vi "FinalizeListGeneration.vi"(8 "error in (no error)":errorcluster, 9 "Root path":path, 10 "CDependencyList in":refnum<class "CDependencyList.lvclass">, 11 "CReporter in":refnum<class "CReporter.lvclass">) -> (0 "error out":errorcluster, 3 "CReporter out":refnum<class "CReporter.lvclass">)   [LabVIEW 2020, in "DependencyInspection.lvlib" / "CReporter.lvclass"]
uses:
  CReporter.lvclass
  CDependencyList/CDependencyList.lvclass
  CReporter.lvclass/CReporter.ctl
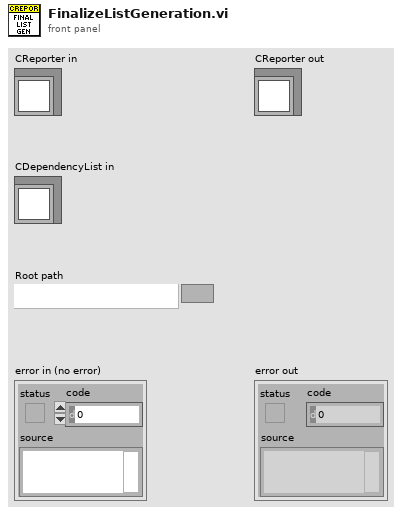
[diagram p1: front panel]
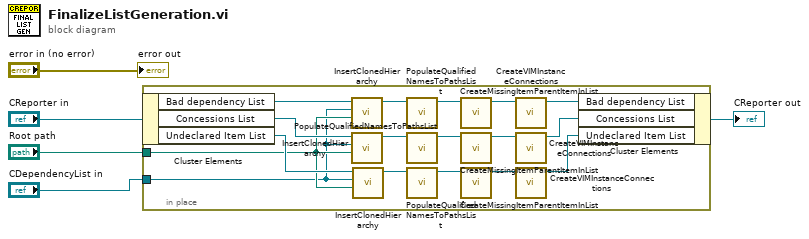
[diagram p0: block diagram]
diagram:
  n1 = in-place {
    in-place-border: "Root path" -> [w7]
    in-place-border: "CDependencyList in" -> [w6]
    n2 = in-place-cluster #1("CReporter in") -> ("Bad dependency List"=w13:refnum<class "CDependencyList.lvclass">, "Concessions List"=w11:refnum<class "CDependencyList.lvclass">, "Undeclared Item List"=w9:refnum<class "CDependencyList.lvclass">)
    n3 = call-dynamic "InsertClonedHierarchy.vi"("Root path"=w7, "Dependency List in"=w6, "CDependencyList in"=w13) -> ("CDependencyList out"=w12:refnum<class "CDependencyList.lvclass">)  [unwired: 7 in, 1 out]
    n4 = call-dynamic "InsertClonedHierarchy.vi"("Root path"=w7, "Dependency List in"=w6, "CDependencyList in"=w11) -> ("CDependencyList out"=w10:refnum<class "CDependencyList.lvclass">)  [unwired: 7 in, 1 out]
    n5 = call-dynamic "InsertClonedHierarchy.vi"("Root path"=w7, "Dependency List in"=w6, "CDependencyList in"=w9) -> ("CDependencyList out"=w8:refnum<class "CDependencyList.lvclass">)  [unwired: 7 in, 1 out]
    n6 = call-dynamic "PopulateQualifiedNamesToPathsList.vi"("CDependencyList in"=w12) -> ("CDependencyList out"=w21:refnum<class "CDependencyList.lvclass">)  [unwired: 9 in, 1 out]
    n7 = call-dynamic "PopulateQualifiedNamesToPathsList.vi"("CDependencyList in"=w10) -> ("CDependencyList out"=w19:refnum<class "CDependencyList.lvclass">)  [unwired: 9 in, 1 out]
    n8 = call-dynamic "PopulateQualifiedNamesToPathsList.vi"("CDependencyList in"=w8) -> ("CDependencyList out"=w17:refnum<class "CDependencyList.lvclass">)  [unwired: 9 in, 1 out]
    n9 = call-dynamic "CreateMissingItemParentItemInList.vi"("CDependencyList in"=w21) -> ("CDependencyList out"=w22:refnum<class "CDependencyList.lvclass">)  [unwired: 9 in, 1 out]
    n10 = call-dynamic "CreateMissingItemParentItemInList.vi"("CDependencyList in"=w19) -> ("CDependencyList out"=w20:refnum<class "CDependencyList.lvclass">)  [unwired: 9 in, 1 out]
    n11 = call-dynamic "CreateMissingItemParentItemInList.vi"("CDependencyList in"=w17) -> ("CDependencyList out"=w18:refnum<class "CDependencyList.lvclass">)  [unwired: 9 in, 1 out]
    n12 = call-dynamic "CreateVIMInstanceConnections.vi"("CDependencyList in"=w22) -> ("CDependencyList out"=w16:refnum<class "CDependencyList.lvclass">)  [unwired: 9 in, 1 out]
    n13 = call-dynamic "CreateVIMInstanceConnections.vi"("CDependencyList in"=w20) -> ("CDependencyList out"=w15:refnum<class "CDependencyList.lvclass">)  [unwired: 9 in, 1 out]
    n14 = call-dynamic "CreateVIMInstanceConnections.vi"("CDependencyList in"=w18) -> ("CDependencyList out"=w14:refnum<class "CDependencyList.lvclass">)  [unwired: 9 in, 1 out]
    n15 = in-place-cluster #1("Bad dependency List"=w16, "Concessions List"=w15, "Undeclared Item List"=w14) -> (→"CReporter out":refnum<class "CReporter.lvclass">)
  }
  "error out" <- "error in (no error)"
